vi "T chart calculations.vi"(0 "Scale Control":T8, 2 "clear chart":bool, 7 "WaveformChart in":refnum<vi>, 11 "T cont":T1={"exec"={"T mode"=enum."Listening to exec", "exec setpoint"=30.0, "reset"=FALSE, "man power"=0.5, "man"=FALSE, "log"=FALSE, "clear"=FALSE}, "T status"={"Control status"=enum."Below Control Band", "Temp"=0.0, "Power"=0.0, "Time in settle band"=0.0, "Settled"=FALSE, "Low"=FALSE, "High"=FALSE, "Setpoint"=30.0, "Control"=FALSE, "In Settle Band"=FALSE}, "T params"={"Setpoint"=50.0, "Control Bandwidth"=4.0, "Integral Time"=30.0, "Int\nON"=TRUE, "Derivative Tme"=0.5, "Der\nON"=TRUE, "Settle Bandwidth"=1.0, "Settle Time"=60.0}, "utility"={"meas index"=300, "wait (ms)"=0, "H Vmax"=8.5, "power out"=0.0, "heat volt out"=0.0, "heat volt in"=0.0, "therm volt"=0.0, "t T P hist"=[], "cont hist"=[]}} {"utility"."therm volt" format="%_6g"; "utility"."heat volt in" format="%_6g"; "utility"."heat volt out" format="%_6g"; "utility"."power out" format="%_6g"; "utility"."H Vmax" format="%_6g"; "exec"."man power" format="%_6g"; "exec"."exec setpoint" format="%_6g"; "T params"."Settle Time" step=1.0; "T params"."Settle Bandwidth" step=0.01; "T params"."Derivative Tme" step=0.01; "T params"."Integral Time" step=1.0; "T params"."Control Bandwidth" step=0.1; "T params"."Setpoint" step=0.1; "T status"."Setpoint" format="%_6g"; "T status"."Power" format="%_6g"; "T status"."Temp" format="%_6g"}) -> (4 "T chart cluster":T9, 15 "Setpoint":dbl)   [LabVIEW 2019]
doc: "This subVI handles the scale change requests for the temeperature chart, and does the calulations for the temperature chart in the bug experiment.\n\nIt scales the power varaible to be normalized to [0,1] on the vertical temp scale dynamicallly. It clears the power history on scale change.\n\nIt also clears the chart on command.\n\nPaul K Dixon\nP3600\nCSUSB Physics"
uses:
  typedefs/scale control.ctl
  typedefs/temp cont cluster.ctl
  typedefs/temp exec cluster.ctl
  typedefs/temp mode enum.ctl
  typedefs/temp indicator.ctl
  typedefs/temp control status.ctl
  typedefs/PID control parameters.ctl
  typedefs/temp cont utility.ctl
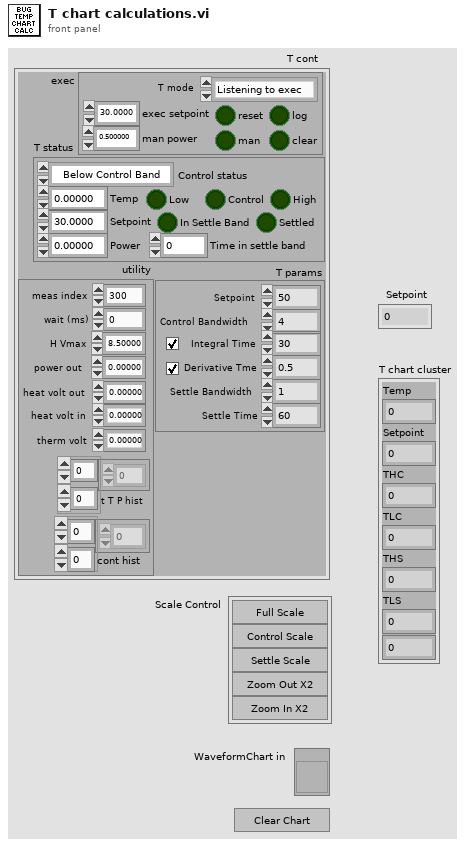
[diagram p1: front panel]
types:
  T1 = typedef "temp cont cluster.ctl" = cluster{"exec":T2, "T status":T4, "T params":T6, "utility":T7}
  T2 = typedef "temp exec cluster.ctl" = cluster{"T mode":T3, "exec setpoint":dbl, "reset":bool, "man power":dbl, "man":bool, "log":bool, "clear":bool}
  T3 = typedef "temp mode enum.ctl" = enum16{"Setting up", "Listening to exec", "Exit"}
  T4 = typedef "temp indicator.ctl" = cluster{"Control status":T5, "Temp":dbl, "Power":dbl, "Time in settle band":dbl, "Settled":bool, "Low":bool, "High":bool, "Setpoint":dbl, "Control":bool, "In Settle Band":bool}
  T5 = typedef "temp control status.ctl" = enum16{"In Settle Band", "In Control Band", "Below Control Band", "Above Control Band"}
  T6 = typedef "PID control parameters.ctl" = cluster{"Setpoint":dbl, "Control Bandwidth":dbl, "Integral Time":dbl, "Int\nON":bool, "Derivative Tme":dbl, "Der\nON":bool, "Settle Bandwidth":dbl, "Settle Time":dbl}
  T7 = typedef "temp cont utility.ctl" = cluster{"meas index":i32, "wait (ms)":i32, "H Vmax":dbl, "power out":dbl, "heat volt out":dbl, "heat volt in":dbl, "therm volt":dbl, "t T P hist":dbl[][], "cont hist":dbl[][]}
  T8 = typedef "scale control.ctl" = cluster{"Full Scale":bool, "Control Scale":bool, "Settle Scale":bool, "Zoom Out X2":bool, "Zoom In X2":bool}
  T9 = cluster{"Temp":dbl, "Setpoint":dbl, "THC":dbl, "TLC":dbl, "THS":dbl, "TLS":dbl, dbl}
  T10 = cluster{"temp out":dbl, dbl, dbl, dbl, dbl, dbl, dbl}[]
  T11 = cluster{"temp out":dbl, dbl, dbl, dbl, dbl, dbl, dbl}
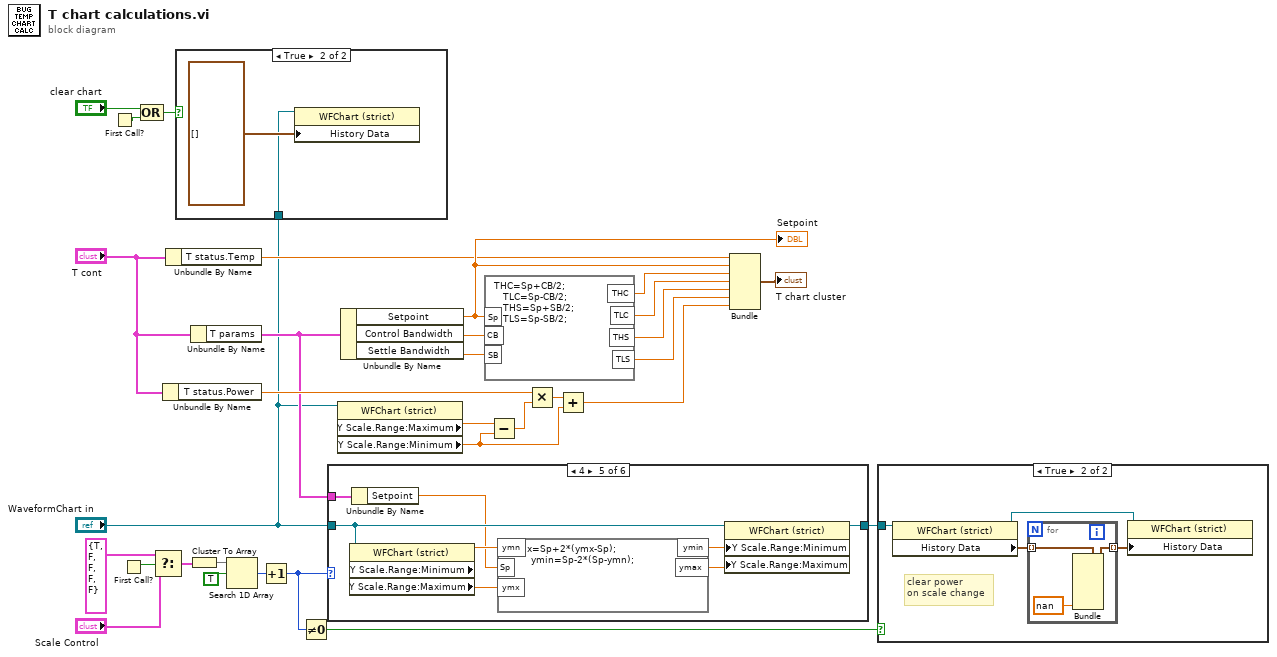
[diagram p0: block diagram]
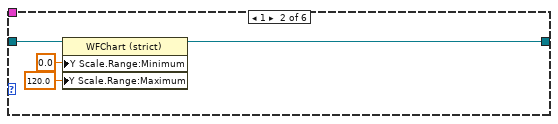
[diagram p5: hidden frame]
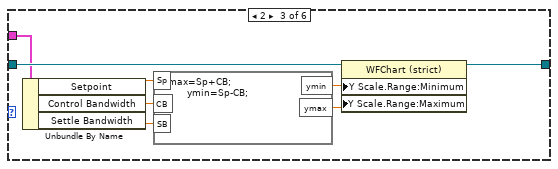
[diagram p6: hidden frame]
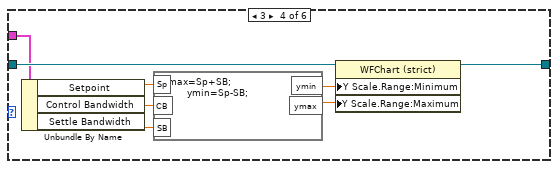
[diagram p7: hidden frame]
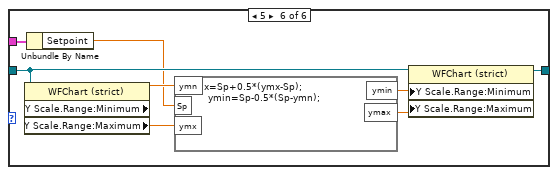
[diagram p8: hidden frame]
diagram:
  n1 = First Call?() -> (First Call?: T/F=w2:bool)
  n2 = First Call?() -> (First Call?: T/F=w8:bool)
  n3 = Compound Arithmetic op=OR("clear chart", w2) -> (w1:bool)
  n4 = Select(t=T8 {"Full Scale"=TRUE, "Control Scale"=FALSE, "Settle Scale"=FALSE, "Zoom Out X2"=FALSE, "Zoom In X2"=FALSE} ("Scale Control"), s=w8, f="Scale Control") -> (s? t:f=w5:T8)
  n5 = Unbundle By Name("T cont") -> ("T status.Power"=w11:dbl)
  n6 = Unbundle By Name("T cont") -> ("T status.Temp"=w9:dbl)
  n7 = case shown="True" w1 {
    tunnel: "WaveformChart in" -> [_ w32]
    frame False {
    }
    frame True {
      n8 = property on="Property Node" class="WFChart (strict)"(reference=w32, "History Data"=T10 []) -> ()  [unwired: 1 in, 2 out]
    }
  }
  n9 = Cluster To Array(cluster=w5) -> (array=w15:bool[])
  n10 = Unbundle By Name("T cont") -> ("T params"=w10:T6)
  n11 = Search 1D Array(1D array=w15, element=TRUE) -> (index of element=w13:i32)  [unwired: 1 out]
  n12 = Increment(x=w13) -> (x+1=w30:i32)
  n13 = Not Equal To 0?(x=w30) -> (x != 0?=w31:bool)
  n14 = case shown="4" w30 {
    tunnel: w10 -> [_ _ w42 w50 w56 w64]
    tunnel: "WaveformChart in" -> [w34 w36 w44 w52 w58 w65]
    tunnel: [w34 w35 w43 w51 w57 w66] -> w29
    frame 0, Default {
    }
    frame 1 {
      n15 = property on="Property Node" class="WFChart (strict)"(reference=w36, "Y Scale.Range:Minimum"=0.0, "Y Scale.Range:Maximum"=120.0) -> (reference out=w35:refnum<vi>)  [unwired: 1 in, 1 out]
    }
    frame 2 {
      n16 = Unbundle By Name(w42) -> ("Setpoint"=w41:dbl, "Control Bandwidth"=w40:dbl, "Settle Bandwidth"=w39:dbl)
      n17 = formula code="ymax=Sp+CB;\n        ymin=Sp-CB;"("Sp"=w41, "CB"=w40, "SB"=w39) -> ("ymax"=w45:dbl, "ymin"=w46:dbl)
      n18 = property on="Property Node" class="WFChart (strict)"(reference=w44, "Y Scale.Range:Minimum"=w46, "Y Scale.Range:Maximum"=w45) -> (reference out=w43:refnum<vi>)  [unwired: 1 in, 1 out]
    }
    frame 3 {
      n19 = Unbundle By Name(w50) -> ("Setpoint"=w49:dbl, "Control Bandwidth"=w48:dbl, "Settle Bandwidth"=w47:dbl)
      n20 = formula code="ymax=Sp+SB;\n        ymin=Sp-SB;"("Sp"=w49, "CB"=w48, "SB"=w47) -> ("ymax"=w53:dbl, "ymin"=w54:dbl)
      n21 = property on="Property Node" class="WFChart (strict)"(reference=w52, "Y Scale.Range:Minimum"=w54, "Y Scale.Range:Maximum"=w53) -> (reference out=w51:refnum<vi>)  [unwired: 1 in, 1 out]
    }
    frame 4 {
      n22 = property on="Property Node" class="WFChart (strict)"(reference=w58) -> ("Y Scale.Range:Minimum"=w60:dbl, "Y Scale.Range:Maximum"=w59:dbl)  [unwired: 1 in, 2 out]
      n23 = Unbundle By Name(w56) -> ("Setpoint"=w55:dbl)
      n24 = formula code="ymax=Sp+2*(ymx-Sp);\n        ymin=Sp-2*(Sp-ymn);"("ymn"=w60, "Sp"=w55, "ymx"=w59) -> ("ymax"=w61:dbl, "ymin"=w62:dbl)
      n25 = property on="Property Node" class="WFChart (strict)"(reference=w58, "Y Scale.Range:Minimum"=w62, "Y Scale.Range:Maximum"=w61) -> (reference out=w57:refnum<vi>)  [unwired: 1 in, 1 out]
    }
    frame 5 {
      n26 = property on="Property Node" class="WFChart (strict)"(reference=w65) -> ("Y Scale.Range:Minimum"=w68:dbl, "Y Scale.Range:Maximum"=w67:dbl)  [unwired: 1 in, 2 out]
      n27 = Unbundle By Name(w64) -> ("Setpoint"=w63:dbl)
      n28 = formula code="ymax=Sp+0.5*(ymx-Sp);\n        ymin=Sp-0.5*(Sp-ymn);"("ymn"=w68, "Sp"=w63, "ymx"=w67) -> ("ymax"=w69:dbl, "ymin"=w70:dbl)
      n29 = property on="Property Node" class="WFChart (strict)"(reference=w65, "Y Scale.Range:Minimum"=w70, "Y Scale.Range:Maximum"=w69) -> (reference out=w66:refnum<vi>)  [unwired: 1 in, 1 out]
    }
  }
  n30 = property class="WFChart (strict)"(reference="WaveformChart in") -> ("Y Scale.Range:Maximum"=w19:dbl, "Y Scale.Range:Minimum"=w18:dbl)  [unwired: 1 in, 2 out]
  n31 = Unbundle By Name(w10) -> ("Setpoint"=w27:dbl, "Control Bandwidth"=w21:dbl, "Settle Bandwidth"=w20:dbl)
  "Setpoint" <- w27
  n32 = formula code="THC=Sp+CB/2;\n   TLC=Sp-CB/2;\n   THS=Sp+SB/2;\n   TLS=Sp-SB/2;"("Sp"=w27, "CB"=w21, "SB"=w20) -> ("THC"=w26:dbl, "TLC"=w24:dbl, "THS"=w25:dbl, "TLS"=w23:dbl)
  n33 = Subtract(x=w19, y=w18) -> (x-y=w16:dbl)
  n34 = Multiply(x=w11, y=w16) -> (x*y=w17:dbl)
  n35 = Add(x=w17, y=w18) -> (x+y=w22:dbl)
  n36 = Bundle("Temp"=w9, "Setpoint"=w27, "THC"=w26, "TLC"=w24, "THS"=w25, "TLS"=w23, w22) -> (→"T chart cluster":T9)  [unwired: 1 out]
  n37 = case shown="True" w31 {
    tunnel: w29 -> [_ w71]
    frame False {
    }
    frame True {
      # "clear power\non scale change"
      n38 = property class="WFChart (strict)"(reference=w71) -> (reference out=w74:refnum<vi>, "History Data"=w72:T10)  [unwired: 1 in, 1 out]
      n39 = for {
        tunnel: w72 -> [w77] mode=indexing
        tunnel: [w76] -> w73 mode=indexing
        n40 = Bundle(cluster=w77, nan) -> (w76:T11)  [unwired: 6 in]
      }
      n41 = property on="Property Node" class="WFChart (strict)"(reference=w74, "History Data"=w73) -> ()  [unwired: 1 in, 2 out]
    }
  }
